vi "ID Query.vi"(8 "error in (no error)":errorcluster, 10 "Node (3)":u8=3 caption="Node" min=3 max=128 step=1, 11 "VISA resource name":refnum<visa-resource-name>) -> (0 "error out":errorcluster, 1 "Modelnumber":string, 2 "Serialnumber":string, 3 "VISA resource name out":refnum<visa-resource-name>, 4 "Device ID number":u32, 6 "Device Type and Description":string)   [LabVIEW 2024, in "Bronkhorst FLOW-BUS.lvlib"]
doc: "This VI Querys the instrument for two values, the Modelnumber and the Serialnumber. These numbers are used to identify the attached instrument."
uses:
  Bronkhorst FLOW-BUS.lvlib
  FLOW-BUS RW.ctl
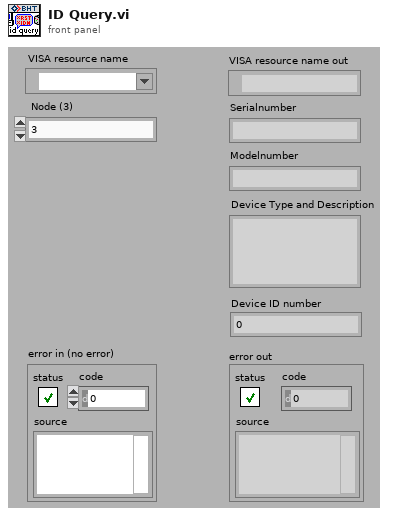
[diagram p1: front panel]
types:
  T1 = enum16{"Character", "Integer", "Float or Long", "String"}
  T2 = typedef "Bronkhorst FLOW-BUS.lvlib/FLOW-BUS RW.ctl" = cluster{"Node Address (3)":u8, "Communication Command":enum16{"Status message", "Send parameter with destination address and 00 response", "Send parameter with destination address", "Request parameter"}, "Process (0)":u16, "Parameter (0)":u16, "Data Type (0: Character)":enum16{"Character", "Integer", "Float or Long", "String"}, "Data for Char, Int, or Long (0)":u32, "Data for Float (0)":sgl, "Data for String":string, "Length of Requested String (0)":u8}
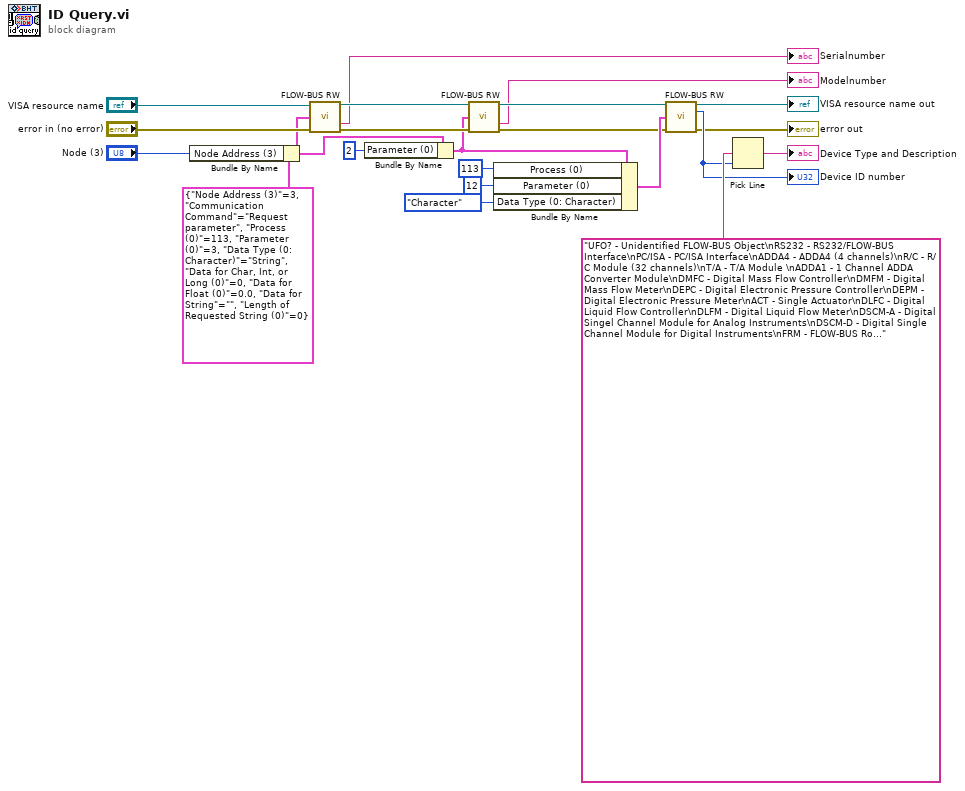
[diagram p0: block diagram]
diagram:
  n1 = Bundle By Name(cluster=T2 {"Node Address (3)"=3, "Communication Command"=enum."Request parameter", "Process (0)"=113, "Parameter (0)"=3, "Data Type (0: Character)"=enum."String", "Data for Char, Int, or Long (0)"=0, "Data for Float (0)"=0.0, "Data for String"="", "Length of Requested String (0)"=0} ("FLOW-BUS Command Settings"), "Node Address (3)"="Node (3)") -> (w3:T2)
  n2 = call "FLOW-BUS RW.vi"("VISA resource name"="VISA resource name", "FLOW-BUS Command Settings"=w3, "error in (no error)"="error in (no error)") -> ("VISA resource name out"=w16:refnum<visa-resource-name>, "Requested String"=→"Serialnumber":string, "error out"=w15:errorcluster)  [unwired: 8 in, 2 out]
  n3 = Bundle By Name(cluster=w3, "Parameter (0)"=u16 2 ("Data for Char or Int")) -> (w11:T2)
  n4 = call "FLOW-BUS RW.vi"("VISA resource name"=w16, "FLOW-BUS Command Settings"=w11, "error in (no error)"=w15) -> ("VISA resource name out"=w8:refnum<visa-resource-name>, "Requested String"=→"Modelnumber":string, "error out"=w9:errorcluster)  [unwired: 8 in, 2 out]
  n5 = Bundle By Name(cluster=w11, "Process (0)"=u16 113 ("Process"), "Parameter (0)"=u16 12 ("Parameter"), "Data Type (0: Character)"=T1."Character" ("Data Type")) -> (w10:T2)
  n6 = call "FLOW-BUS RW.vi"("VISA resource name"=w8, "FLOW-BUS Command Settings"=w10, "error in (no error)"=w9) -> ("VISA resource name out"=→"VISA resource name out":refnum<visa-resource-name>, "Requested Char, Int or Long"=w20:u32, "error out"=→"error out":errorcluster)  [unwired: 8 in, 2 out]
  "Device ID number" <- w20
  n7 = Pick Line(multi-line string="UFO? - Unidentified FLOW-BUS Object\nRS232 - RS232/FLOW-BUS Interface\nPC/ISA - PC/ISA Interface\nADDA4 - ADDA4 (4 channels)\nR/C - R/C Module (32 channels)\nT/A - T/A Module \nADDA1 - 1 Channel ADDA Converter Module\nDMFC - Digital Mass Flow Controller\nDMFM - Digital Mass Flow Meter\nDEPC - Digital Electronic Pressure Controller\nDEPM - Digital Electronic Pressure Meter\nACT - Single Actuator\nDLFC - Digital Liquid Flow Controller\nDLFM - Digital Liquid Flow Meter\nDSCM-A - Digital Singel Channel Module for Analog Instruments\nDSCM-D - Digital Single Channel Module for Digital Instruments\nFRM - FLOW-BUS Rotor Meter (calibration-instrument)\nFTM - FLOW-BUS Turbine Meter (calibration-instrument)\nFPP - FLOW-BUS Piston Prover/Tube (calibration-instrument)\nF/A - Special Version of T/A Module\nDSCM-E - Digital Single Channel Module for Evaporators\nDSCM-C - Digital Single Channel Module for Calibrators\nDDCM-A - Digital Dual Channel Module for Analog Instruments\nDMCM-D - Digital Multi Channel Module for Digital Instruments\nPRODPS - PROFIBUS DP / FLOW-BUS -Slave Interface\nFCM - FLOW-BUS Coriolis Meter\nFBI - FLOW-BUS Balance Interface\nCORIFC - (mini) CORI-FLOW Controller\nCORIFM - (mini) CORI-FLOW Meter\nFICC - FLOW-BUS Interface Climate Control\nIFI - Instrument FLOW-BUS Interface\nKFI - Keithly FLOW-BUS Interface\nFSI - FLOW-BUS Switch Interface\nMSCI - Multi Sensor/Controller Interface\nAPP-D - Active Piston Prover (calibration-instrument)\nLFI - Leak Tester FLOW-BUS Interface", line index=w20) -> (output string=→"Device Type and Description":string)  [unwired: 1 in]
